vi "Write Linear PID Tuning.vi"(8 "error in (no error)":errorcluster, 10 "Linear PID Tuning":T2, 11 "Supervisor in":refnum<class "Supervisor.lvclass">) -> (0 "error out":errorcluster, 3 "Supervisor out":refnum<class "Supervisor.lvclass">)   [LabVIEW 2014, in "Supervisor.lvclass"]
uses:
  Supervisor.lvclass
  <vilib>/Analysis/Matrix/Datatypes/RealMatrix.ctl
  Supervisor.lvclass/Supervisor.ctl
  <vilib>/Analysis/Matrix/NI_Matrix.lvlib
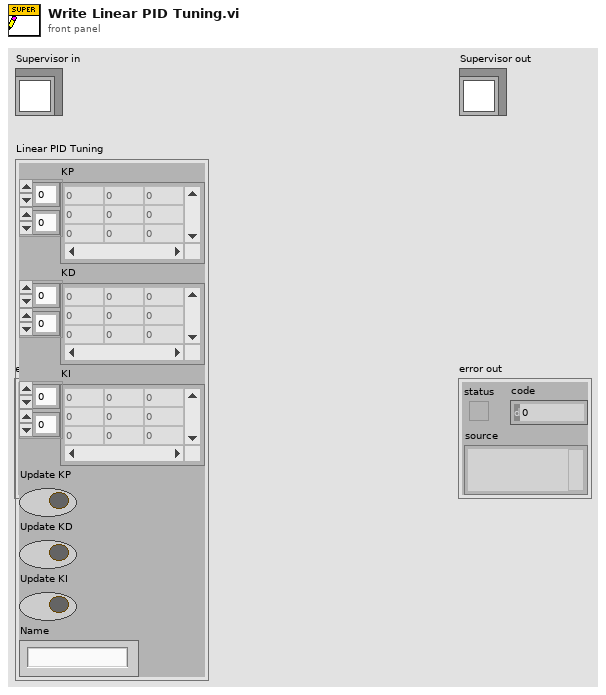
[diagram p1: front panel]
types:
  T1 = typedef "NI_Matrix.lvlib/RealMatrix.ctl" = dbl[][]
  T2 = cluster{"KP":T1, "KD":T1, "KI":T1, "Update KP":bool, "Update KD":bool, "Update KI":bool, "Name":string}
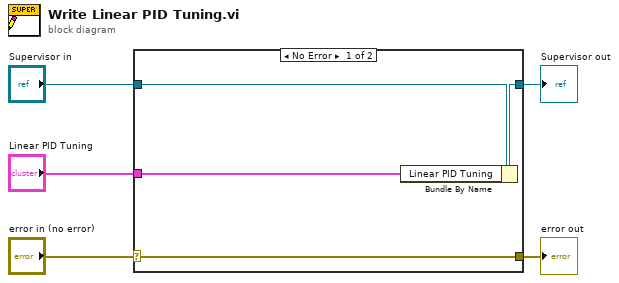
[diagram p0: block diagram]
diagram:
  n1 = case shown="No Error" "error in (no error)" {
    selector: "error in (no error)" -> [w9 w10]
    tunnel: [w9 w10] -> w4
    tunnel: [w7 w11] -> w2
    tunnel: "Supervisor in" -> [w8 w11]
    tunnel: "Linear PID Tuning" -> [w6 _]
    frame No Error {
      n2 = Bundle By Name(cluster=w8, "Linear PID Tuning"=w6) -> (w7:refnum<class "Supervisor.lvclass">)
    }
    frame Error {
    }
  }
  "error out" <- w4
  "Supervisor out" <- w2
